vi "Get Endpoint Configuration.vi"(8 "error in":errorcluster, 10 "endpoint":string, 11 "endpoint configuration in":T2 format="%.0x") -> (0 "error out":errorcluster, 2 "configuration":T1, 3 "endpoint configuration out":T2 format="%.0x")   [LabVIEW 2020, in "SLSC Switch Scripting.lvlib"]
doc: "Returns the configuration for one endpoint."
uses:
  SLSC Switch Scripting.lvlib
  <vilib>/NI VeriStand/Custom Device API/Custom Device Item Ref.ctl
  Shared/Endpoint Configuration Enum.ctl
  <vilib>/NI VeriStand/Custom Device API/Get Item Property (String).vi
  <vilib>/NI VeriStand/Custom Device API/Custom Device API.lvlib
  Dependencies.llb/SLSC Switch Shared.lvlib
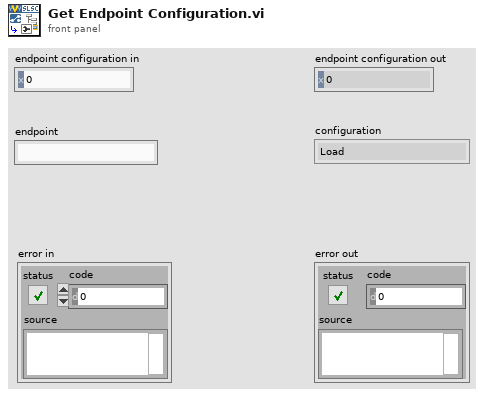
[diagram p1: front panel]
types:
  T1 = typedef "SLSC Switch Shared.lvlib/Endpoint Configuration Enum.ctl" = enum16{"Load", "Source", "Configuration"}
  T2 = typedef "Custom Device API.lvlib/Custom Device Item Ref.ctl" = u64
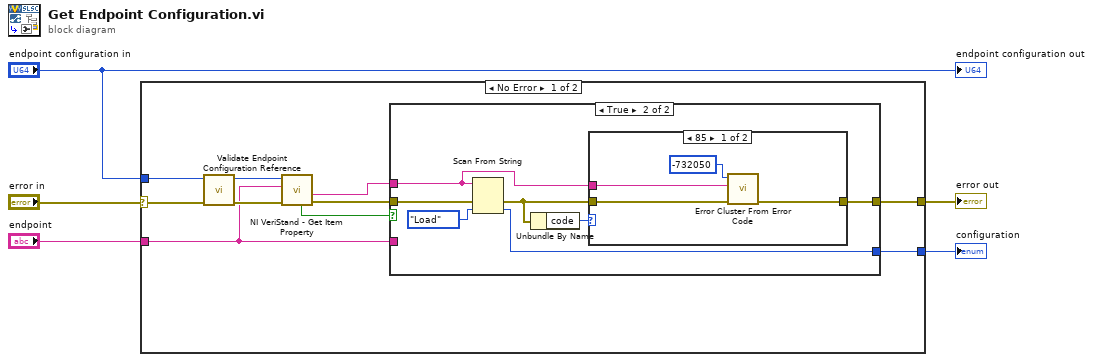
[diagram p0: block diagram]
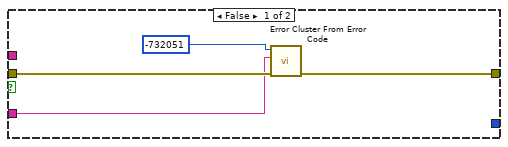
[diagram p2: hidden frame]
diagram:
  n1 = case shown="No Error" "error in" {
    selector: "error in" -> [w15 w32]
    tunnel: [w11 _] -> w4
    tunnel: [w10 w32] -> w3
    tunnel: "endpoint configuration in" -> [w8 _]
    tunnel: "endpoint" -> [w6 _]
    frame No Error {
      n2 = call "Validate Endpoint Configuration Reference.vi"("error in"=w15, "endpoint configuration in"=w8) -> ("error out"=w9:errorcluster, "endpoint configuration out"=w7:T2)  [unwired: 8 in]
      n3 = call-poly <vilib>:"NI VeriStand - Get Item Property.vi"("error in (no error)"=w9, "Property Name"=w6, "Item Ref in"=w7) -> ("error out"=w13:errorcluster, "Value"=w12:string, "Found?"=w14:bool)  [unwired: 5 in, 1 out]
      n4 = case shown="True" w14 {
        tunnel: w13 -> [w18 w24]
        tunnel: w12 -> [_ w22]
        tunnel: [_ w26] -> w11
        tunnel: [w17 w23] -> w10
        tunnel: w6 -> [w16 _]
        frame False {
          n5 = call <vilib>:"Error Cluster From Error Code.vi"("error in (no error)"=w18, "error message (\"\")"=w16, "error code (0)"=-732051) -> ("error out"=w17:errorcluster)  [unwired: 6 in]
        }
        frame True {
          n6 = Scan From String(input string=w22, error in=w24, default 1=Endpoint_Configuration_Enum."Load" ("Configuration Type")) -> (error out=w21:errorcluster, output 1=w26:T1)  [unwired: 2 in, 2 out]
          n7 = Unbundle By Name(w21) -> ("code"=w20:i32)
          n8 = case shown="85" w20 {
            tunnel: [w29 w31] -> w23
            tunnel: w22 -> [w27 _]
            tunnel: w21 -> [w28 w31]
            frame 85 {
              n9 = call <vilib>:"Error Cluster From Error Code.vi"("error in (no error)"=w28, "error message (\"\")"=w27, "error code (0)"=-732050) -> ("error out"=w29:errorcluster)  [unwired: 6 in]
            }
            frame Default {
            }
          }
        }
      }
    }
    frame Error {
    }
  }
  "error out" <- w3
  "configuration" <- w4
  "endpoint configuration out" <- "endpoint configuration in"
